vi "CTL_Load.vi"(0 "File Path":path, 3 "Error In":errorcluster) -> (7 "Data":cluster{"Name":string, "Variant Data":variant}[](array[cluster]), 10 "Error Out":errorcluster)   [LabVIEW 2019]
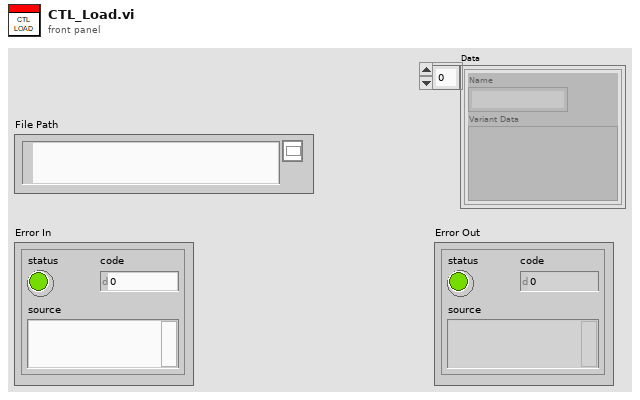
[diagram p1: front panel]
types:
  T1 = enum16{"open", "replace", "create", "open or create", "replace or create", "replace or create with confirmation"}
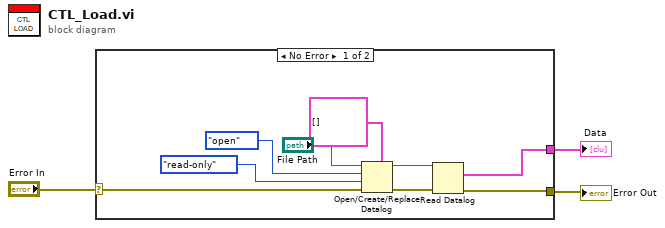
[diagram p0: block diagram]
diagram:
  n1 = case shown="No Error" "Error In" {
    selector: "Error In" -> [w5 w13]
    tunnel: [w7 w13] -> w2
    tunnel: [w4 _] -> w1
    frame No Error {
      n2 = Open/Create/Replace Datalog(5:cluster{"Name":string, "Variant Data":variant}[] [] ("Control Value:Get All"), 8:w5, 9:enum16{"read/write", "read-only", "write-only"}."read-only" ("access (0:read/write)"), 10:T1."open" ("operation (0:open)"), 11:"File Path") -> (0:w8:errorcluster, 3:w9:refnum<k1>)  [unwired: 1 in, 1 out]
      n3 = Read Datalog(4:w8, 7:w9) -> (0:w7:errorcluster, 2:w4:cluster{"Name":string, "Variant Data":variant}[])  [unwired: 1 in, 1 out]
    }
    frame Error {
    }
  }
  "Error Out" <- w2
  "Data" <- w1
